vi "Is DAQ server running.vi"(11 "error in (no error)":errorcluster) -> (8 "Running?":bool, 15 "error out":errorcluster)   [LabVIEW 2015]
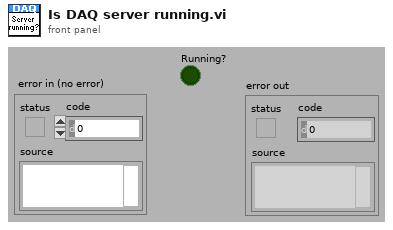
[diagram p1: front panel]
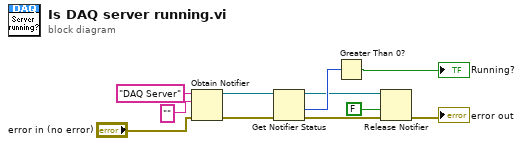
[diagram p0: block diagram]
diagram:
  n1 = Obtain Notifier(name (unnamed)="DAQ Server", notification data type="", error in (no error)="error in (no error)") -> (notifier out=w6:refnum<notifier>, error out=w5:errorcluster)  [unwired: 1 in, 1 out]
  n2 = Get Notifier Status(notifier=w6, error in (no error)=w5) -> (notifier out=w2:refnum<notifier>, # waiting=w4:i32, error out=w1:errorcluster)  [unwired: 2 out]
  n3 = Greater Than 0?(x=w4) -> (x > 0?=→"Running?":bool)
  n4 = Release Notifier(notifier=w2, force destroy? (F)=FALSE, error in (no error)=w1) -> (error out=→"error out":errorcluster)  [unwired: 2 out]
